vi "Temperature Chamber Main.vi"() -> ()   [LabVIEW 2015]
doc: "This application launches and executes the Tag Bus Data framework configuration for the specified target alias. This is a simple example of the framework API functions, but may also be a suitable starting point for a Host UI or Thick Client that is running a local version of the framework."
uses:
  <vilib>/NI/Module Execution Interface/Engine Runtime/Execution States.ctl
  <vilib>/NI/Module Execution Interface/Engine Runtime/Fault.ctl
  <vilib>/NI/Tag Bus Module Framework/runtime/error classification.ctl
  <vilib>/NI/Module Execution Interface/Engine Runtime/Engine Runtime Interface.lvclass
  <vilib>/NI/DCAF/Tag Editor Core/Framework Configuration Classes/target runtime/PL_Target Runtime.lvclass
  <vilib>/NI/Tag Bus Module Framework/runtime/TBM module execution interface.lvclass
panel:
  in  "Target Alias":string="PC"
  out "engine status":T4(array[cluster])
  in  "Configration File Path":path=path "C:/Users/SE_User/Desktop/DCAF HO2/Excercise/Temperature Controller/TemperatureChamber.pcfg"
  in  "stop":bool
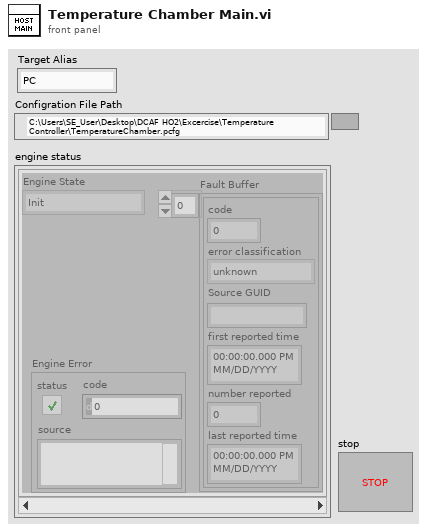
[diagram p1: front panel]
types:
  T1 = typedef "Engine Runtime Interface.lvclass/Execution States.ctl" = enum16{"Init", "Pre-Operational", "Safe-Operational", "Operational", "Stopped"}
  T2 = typedef "Engine Runtime Interface.lvclass/Fault.ctl" = cluster{"code":i32, "error classification":T3, "Source GUID":string, "first reported time":timestamp, "number reported":u32, "last reported time":timestamp}
  T3 = typedef "TBM module execution interface.lvclass/error classification.ctl" = enum16{"unknown", "none", "trivial", "recoverable", "critical"}
  T4 = cluster{"Engine State":T1, "Fault Buffer":T2[], "Engine Error":errorcluster}[]
  T5 = cluster{"Engine State":T1, "faults":T2[], "Engine Error":errorcluster}
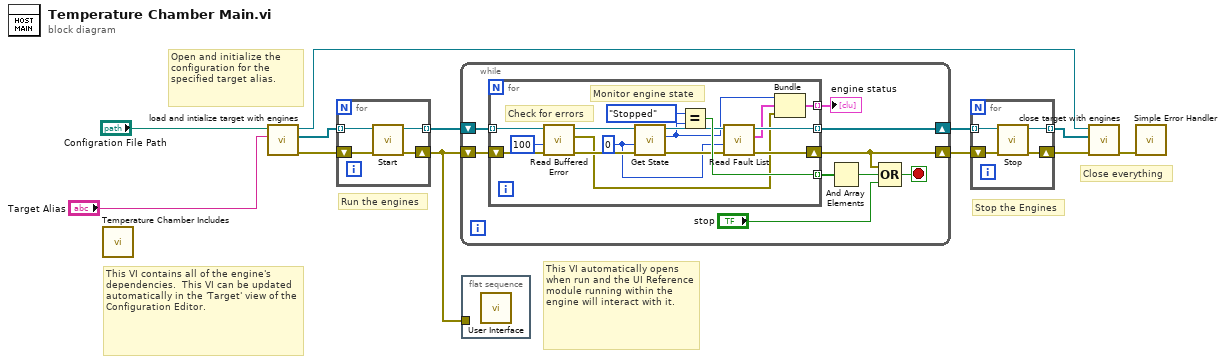
[diagram p0: block diagram]
diagram:
  # "Open and initialize the configuration for the specified target alias."
  # "Close everything"
  # "Stop the Engines"
  # "This VI contains all of the engine's dependencies.  This VI can be updated automatically in the 'Target' view of the Configuration Editor."
  # "This VI automatically opens when run and the UI Reference module running within the engine will interact with it."
  # "Run the engines"
  n1 = call "Temperature Chamber Includes.vi"() -> ()  [unwired: 12 in]
  n2 = call <vilib>:"load and intialize target with engines.vi"("target alias"="Target Alias", "file path"="Configration File Path") -> ("error out"=w8:errorcluster, "engine runtime interfaces"=w7:refnum<class "Engine Runtime Interface.lvclass">[], "target runtime"=w4:refnum<class "PL_Target Runtime.lvclass">)  [unwired: 7 in]
  n3 = for {
    tunnel: [w16] -> w12 mode=indexing
    tunnel: w7 -> [w13] mode=indexing
    shift-right: [w15] -> w9
    shift-left: w8 -> [w14]
    n4 = call-dynamic "Start.vi"("error in"=w14, "Engine Runtime Interface in"=w13) -> ("error out"=w15:errorcluster, "Engine Runtime Interface out"=w16:refnum<class "Engine Runtime Interface.lvclass">)  [unwired: 8 in]
  }
  n5 = while {
    shift-right: [w23] -> w11
    shift-left: w12 -> [w25]
    shift-right: [w20] -> w10
    shift-left: w9 -> [w24]
    stop <- w21 stop-if-true
    n6 = for {
      tunnel: w25 -> [w41] mode=indexing
      tunnel: [w32] -> w23 mode=indexing
      tunnel: [w36] -> w18 mode=indexing
      shift-right: [w31] -> w20
      shift-left: w24 -> [w40]
      tunnel: [w26] -> w19 mode=indexing
      w30 = 0 ("timeout (-1)")
      # "Monitor engine state"
      # "Check for errors"
      n7 = call-dynamic "Read Buffered Error.vi"("error in"=w40, "timeout in ms (0)"=100, "Engine Runtime Interface in"=w41) -> ("error out"=w38:errorcluster, "Engine Error"=w27:errorcluster, "Engine Runtime Interface out"=w39:refnum<class "Engine Runtime Interface.lvclass">)  [unwired: 6 in]
      n8 = call-dynamic "Get State.vi"("error in"=w38, "timeout (-1)"=w30, "Engine Runtime Interface in"=w39) -> ("error out"=w34:errorcluster, "Engine State"=w29:T1, "Engine Runtime Interface out"=w33:refnum<class "Engine Runtime Interface.lvclass">)  [unwired: 6 in]
      n9 = Equal?(x=Execution_States."Stopped" ("Engine State"), y=w29) -> (x = y?=w36:bool)
      n10 = call-dynamic "Read Fault List.vi"("error in"=w34, "timeout (-1)"=w30, "Engine Runtime Interface in"=w33) -> ("error out"=w31:errorcluster, "faults"=w28:T2[], "Engine Runtime Interface out"=w32:refnum<class "Engine Runtime Interface.lvclass">)  [unwired: 6 in]
      n11 = Bundle("Engine State"=w29, "faults"=w28, "Engine Error"=w27) -> (w26:T5)  [unwired: 1 in]
    }
    "engine status" <- w19
    n12 = And Array Elements(Boolean array=w18) -> (logical AND=w17:bool)
    n13 = Compound Arithmetic op=OR(w20, w17, "stop") -> (w21:bool)
  }
  n14 = flat-sequence {
    tunnel: w9 -> [_]
    frame #0 {
      n15 = call "User Interface.vi"() -> ()  [unwired: 12 in]
    }
  }
  n16 = for {
    tunnel: w11 -> [w45] mode=indexing
    shift-right: [w42] -> w3
    shift-left: w10 -> [w44]
    tunnel: [w43] -> w5 mode=indexing
    n17 = call-dynamic "Stop.vi"("error in"=w44, "Engine Runtime Interface in"=w45) -> ("error out"=w42:errorcluster, "Engine Runtime Interface out"=w43:refnum<class "Engine Runtime Interface.lvclass">)  [unwired: 8 in]
  }
  n18 = call <vilib>:"close target with engines.vi"("error in"=w3, "Engine Runtime Interfaces"=w5, "Target Runtime"=w4) -> ("error out"=w2:errorcluster)  [unwired: 8 in]
  n19 = call <vilib>:"Simple Error Handler.vi"("error in (no error)"=w2) -> ()  [unwired: 4 in, 5 out]
